vi "DBSqlSelectToArray.vi"   [LabVIEW 2011]
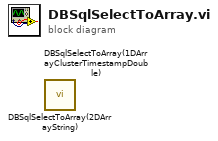
[diagram p0: block diagram]
diagram:
  n1 = call "DBSqlSelectToArray(2DArrayString).vi"() -> ()  [unwired: 10 in, 2 out]
  n2 = call "DBSqlSelectToArray(1DArrayClusterTimestampDouble).vi"() -> ()  [unwired: 10 in, 2 out]
